vi "mod1.vi"() -> ()   [LabVIEW 2016]
uses:
  <vilib>/myRIO/Instrument Drivers/Onboard IO/DIO/vis/Read.vi
  <vilib>/myRIO/Common/Instrument Driver Framework/myRIO v1.0/UART/vis/myRIO v1.0 Close UART.vi
  <vilib>/myRIO/Instrument Drivers/Onboard IO/DIO/vis/Smart Open.vi
  <vilib>/Utility/error.llb/Error Cluster From Error Code.vi
  <vilib>/myRIO/Common/Instrument Driver Framework/myRIO v1.0/DIO/vis/myRIO v1.0 Read DIO.vi
  <vilib>/myRIO/Common/Instrument Driver Framework/Utilities/vis/FPGA Ref Manager.vi
  <vilib>/myRIO/Common/Instrument Driver Framework/myRIO v1.0/myRIO v1.0 Reset FPGA.vi
  <vilib>/myRIO/Common/Instrument Driver Framework/myRIO v1.0/IRQ/vis/myRIO v1.0 IRQ Info FGV.vi
  <vilib>/myRIO/Common/Instrument Driver Framework/myRIO v1.0/IRQ/vis/myRIO v1.0 Timer IRQ Info FGV.vi
  <vilib>/myRIO/Common/Instrument Driver Framework/myRIO v1.0/IRQ/vis/myRIO v1.0 ISR Agent.vi
  <vilib>/myRIO/Instrument Drivers/Utilities/Utilities.lvlib
panel:
  out "unsigned integer":u8
  out "A/DIO state":bool[](array[boolean])
  out "B/DIO state":bool[](array[boolean])
  in  "[ESC]":bool
  # "DIP switches demo"
  # "Rotary DIP"
  # "8-switch DIP"
  # "3       2       1       0"
  # "7       6       5       4       3       2       1       0"
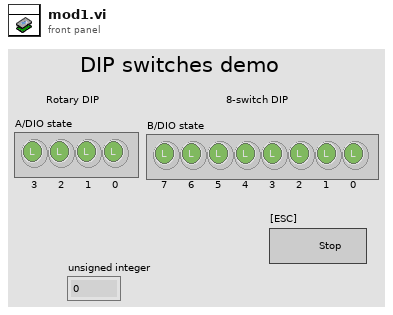
[diagram p1: front panel]
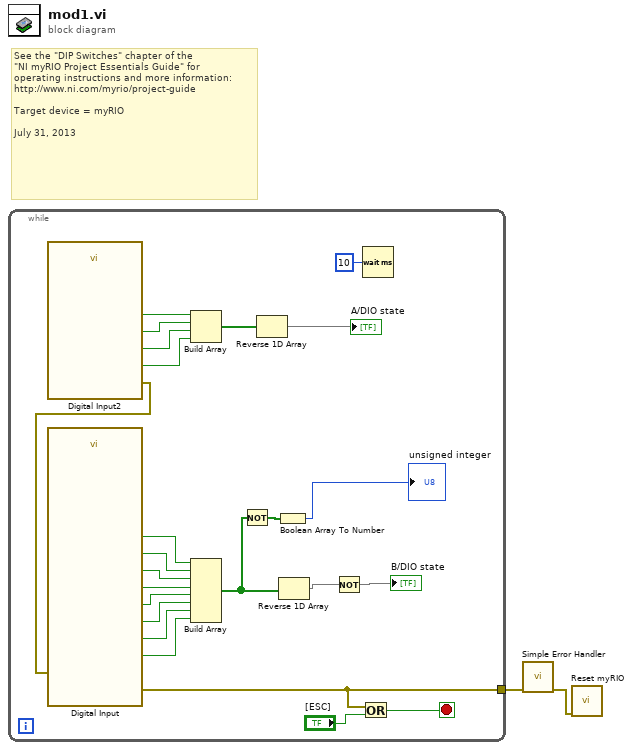
[diagram p0: block diagram]
diagram:
  # "See the \"DIP Switches\" chapter of the \n\"NI myRIO Project Essentials Guide\" for\noperating instructions and more information: \nhttp://www.ni.com/myrio/project-guide\n\nTarget device = myRIO\n\nJuly 31, 2013"
  n1 = while {
    tunnel: [w23] -> w2
    stop <- w26 stop-if-true
    n2 = call "Digital Input2"() -> ("A/DIO0 (Pin 11)"=w10:bool, "A/DIO1 (Pin 13)"=w11:bool, "A/DIO2 (Pin 15)"=w12:bool, "A/DIO3 (Pin 17)"=w13:bool, "error out"=w8:errorcluster)  [unwired: 23 in]
    n3 = call "Digital Input"("error in (no error)"=w8) -> ("B/DIO6 (Pin 23)"=w16:bool, "B/DIO7 (Pin 25)"=w15:bool, "B/DIO0 (Pin 11)"=w22:bool, "B/DIO1 (Pin 13)"=w21:bool, "B/DIO2 (Pin 15)"=w20:bool, "B/DIO3 (Pin 17)"=w19:bool, "B/DIO4 (Pin 19)"=w18:bool, "B/DIO5 (Pin 21)"=w17:bool, "error out"=w23:errorcluster)  [unwired: 18 in]
    n4 = Build Array "Build Array"(w10, w11, w12, w13) -> (w14:bool[])
    n5 = Build Array "Build Array"(w22, w21, w20, w19, w18, w17, w16, w15) -> (w4:bool[])
    n6 = Not(x=w4) -> (.not. x?=w3:bool[])
    n7 = Reverse 1D Array(array=w14) -> (reversed array=→"A/DIO state":bool[])
    n8 = Boolean Array To Number(Boolean array=w3) -> (number=→"unsigned integer":u32)
    n9 = Reverse 1D Array(array=w4) -> (reversed array=w7:bool[])
    n10 = Not(x=w7) -> (.not. x?=→"B/DIO state":bool[])
    n11 = Or(x=w23, y="[ESC]") -> (x .or. y?=w26:bool)
    n12 = Wait (ms)(milliseconds to wait=u32 10) -> ()  [unwired: 1 out]
  }
  n13 = call <vilib>:"Simple Error Handler.vi"("error in (no error)"=w2) -> ("error out"=w1:errorcluster)  [unwired: 4 in, 4 out]
  n14 = call <vilib>:"Reset myRIO.vi"("error in (no error)"=w1) -> ()  [unwired: 10 in, 1 out]
